vi "Shared Variables CD 2.0 Initialization VI.vi"(8 "error in (no error)":errorcluster, 10 "Custom XML":string, 11 "Device Item Ref in":T1 format="%.0x") -> (0 "error out":errorcluster, 3 "Device Item Ref out":T1 format="%.0x")   [LabVIEW 2020, in "Shared Variables CD 2.0 Configuration.lvlib"]
uses:
  Shared Variables CD 2.0 Configuration.lvlib
  <vilib>/NI VeriStand/Custom Device API/Custom Device Item Ref.ctl
  <vilib>/NI VeriStand/Custom Device API/Custom Device Channel.ctl
  <vilib>/NI VeriStand/Custom Device API/Custom Device Channel Type.ctl
  Shared/Shared Variables CD 2.0 GUID Lookup.vi
  Shared/SV Global.vi
  <vilib>/NI VeriStand/Custom Device API/Custom Device API.lvlib
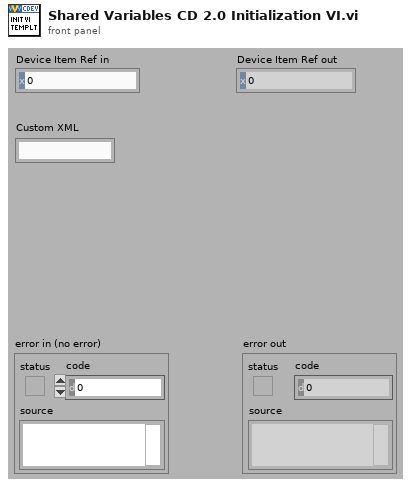
[diagram p1: front panel]
types:
  T1 = typedef "Custom Device API.lvlib/Custom Device Item Ref.ctl" = u64
  T2 = typedef "Custom Device API.lvlib/Custom Device Channel.ctl" = cluster{"Type":T3, "Units":string, "Default Value":dbl, "Faultable":bool, "Scalable":bool}
  T3 = typedef "Custom Device API.lvlib/Custom Device Channel Type.ctl" = enum16{"Input", "Output"}
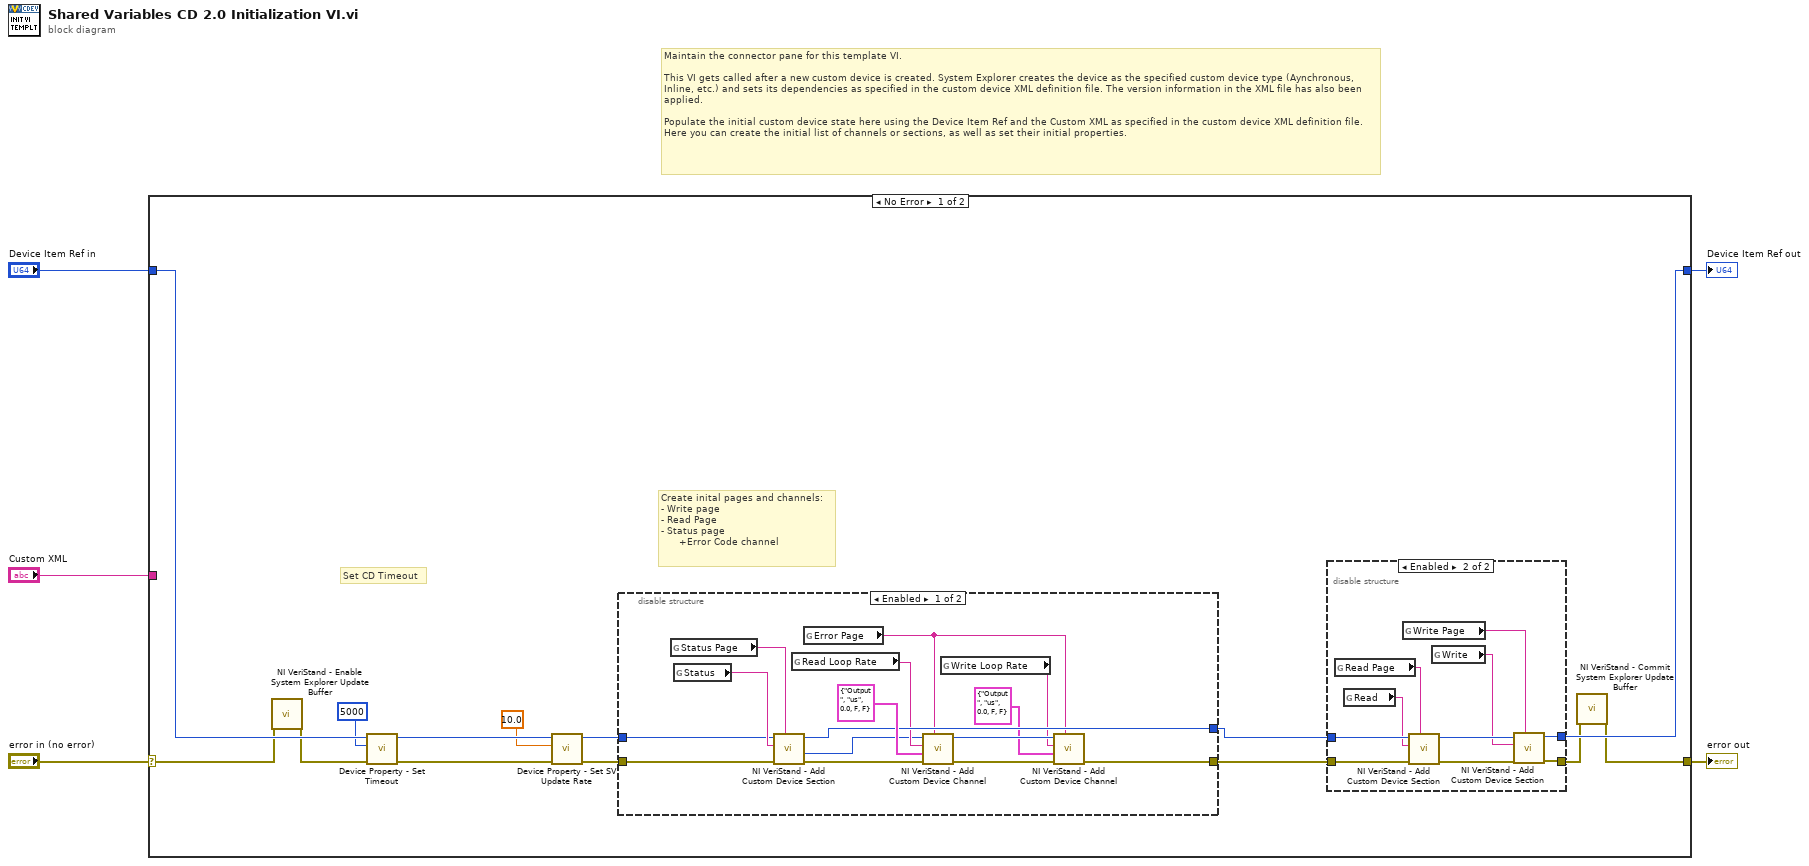
[diagram p0: block diagram]
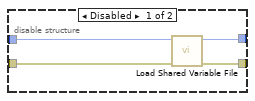
[diagram p3: hidden frame]
diagram:
  # "Maintain the connector pane for this template VI.\n\nThis VI gets called after a new custom device is created. System Explorer creates the device as the specified custom device type (Aynchronous, Inline, etc.) and sets its dependencies as specified in the custom device XML definition file. The version information in the XML file has also been applied.\n\nPopulate the initial custom device state here using the Device Item Ref and the Custom XML as specified in the custom device XML definition file. Here you can create the initial list of channels or sections, as well as set their initial properties."
  n1 = case shown="No Error" "error in (no error)" {
    selector: "error in (no error)" -> [w7 w52]
    tunnel: [w8 w52] -> w5
    tunnel: [w18 w51] -> w3
    tunnel: "Device Item Ref in" -> [w19 w51]
    tunnel: "Custom XML" -> [_ _]
    frame No Error {
      # "Set CD Timeout"
      # "Create inital pages and channels:\n- Write page\n- Read Page\n- Status page\n      +Error Code channel"
      n2 = call <vilib>:"NI VeriStand - Enable System Explorer Update Buffer.vi"("error in (no error)"=w7) -> ("error out"=w6:errorcluster)  [unwired: 10 in]
      n3 = call "Device Property - Set Timeout.vi"("error in (no error)"=w6, "Timout"=5000 ("IP Address"), "Device Ref in"=w19) -> ("error out"=w14:errorcluster, "Device Ref out"=w11:T1)  [unwired: 7 in]
      n4 = call "Device Property - Set SV Update Rate.vi"("error in (no error)"=w14, "Update Rate (ms)"=10.0 ("Value"), "Device Ref in"=w11) -> ("error out"=w13:errorcluster, "Item Ref out"=w12:T1)  [unwired: 7 in]
      n5 = disable-structure shown="Enabled" {
        disable-tunnel: [w33 w36] -> w16
        disable-tunnel: [w24 w35] -> w15
        disable-tunnel: w13 -> [w27 w35]
        disable-tunnel: w12 -> [w26 w36]
        frame Enabled {
          n6 = global read "Shared Variables CD 2.0 GUID Lookup.vi" "Status Page"() -> (w29:string)
          n7 = global read "SV Global.vi" "Status"() -> (w28:string)
          n8 = call <vilib>:"NI VeriStand - Add Custom Device Section.vi"("GUID (Default Section)"=w29, "error in (no error)"=w27, "Section Name"=w28, "Parent Ref in"=w26) -> ("error out"=w31:errorcluster, "Section Ptr"=w30:T1, "Parent Ref out"=w33:T1)  [unwired: 4 in, 1 out]
          n9 = global read "SV Global.vi" "Read Loop Rate"() -> (w32:string)
          n10 = global read "Shared Variables CD 2.0 GUID Lookup.vi" "Error Page"() -> (w21:string)
          n11 = call <vilib>:"NI VeriStand - Add Custom Device Channel.vi"("GUID (Default Channel)"=w21, "error in (no error)"=w31, "Channel"=T2 {"Type"=enum."Output", "Units"="us", "Default Value"=0.0, "Faultable"=FALSE, "Scalable"=FALSE}, "Channel Name"=w32, "Parent Ref in"=w30) -> ("error out"=w25:errorcluster, "Parent Ref out"=w23:T1)  [unwired: 3 in, 2 out]
          n12 = global read "SV Global.vi" "Write Loop Rate"() -> (w22:string)
          n13 = call <vilib>:"NI VeriStand - Add Custom Device Channel.vi"("GUID (Default Channel)"=w21, "error in (no error)"=w25, "Channel"=T2 {"Type"=enum."Output", "Units"="us", "Default Value"=0.0, "Faultable"=FALSE, "Scalable"=FALSE}, "Channel Name"=w22, "Parent Ref in"=w23) -> ("error out"=w24:errorcluster)  [unwired: 3 in, 3 out]
        }
        frame Disabled {
        }
      }
      n14 = disable-structure shown="Enabled" {
        disable-tunnel: [w40 w47] -> w18
        disable-tunnel: [w39 w45] -> w9
        disable-tunnel: w16 -> [w38 w50]
        disable-tunnel: w15 -> [w37 w49]
        frame Disabled {
          n15 = call "Load Shared Variable File.vi"("error in"=w37, "Device Ref in"=w38) -> ("error out"=w39:errorcluster, "Device Ref out"=w40:T1)  [unwired: 8 in]
        }
        frame Enabled {
          n16 = global read "Shared Variables CD 2.0 GUID Lookup.vi" "Read Page"() -> (w44:string)
          n17 = global read "SV Global.vi" "Read"() -> (w41:string)
          n18 = global read "Shared Variables CD 2.0 GUID Lookup.vi" "Write Page"() -> (w43:string)
          n19 = call <vilib>:"NI VeriStand - Add Custom Device Section.vi"("GUID (Default Section)"=w44, "error in (no error)"=w49, "Section Name"=w41, "Parent Ref in"=w50) -> ("error out"=w46:errorcluster, "Parent Ref out"=w48:T1)  [unwired: 4 in, 2 out]
          n20 = global read "SV Global.vi" "Write"() -> (w42:string)
          n21 = call <vilib>:"NI VeriStand - Add Custom Device Section.vi"("GUID (Default Section)"=w43, "error in (no error)"=w46, "Section Name"=w42, "Parent Ref in"=w48) -> ("error out"=w45:errorcluster, "Parent Ref out"=w47:T1)  [unwired: 4 in, 2 out]
        }
      }
      n22 = call <vilib>:"NI VeriStand - Commit System Explorer Update Buffer.vi"("error in (no error)"=w9) -> ("error out"=w8:errorcluster)  [unwired: 10 in]
    }
    frame Error {
    }
  }
  "error out" <- w5
  "Device Item Ref out" <- w3
